vi "Setup Displacement.vi"(8 "error in (no error)":errorcluster, 10 "Model in":refnum<class "Model.lvclass">, 11 "Boot Loader in":refnum<class "Boot Loader.lvclass">) -> (0 "error out":errorcluster, 2 "Model out":refnum<class "Model.lvclass">, 3 "Boot Loader out":refnum<class "Boot Loader.lvclass">)   [LabVIEW 2016, in "Boot Loader.lvclass"]
uses:
  Boot Loader.lvclass
  Model/Model.lvclass
  Common_SerialProtocols/SerialProtocol/SerialReal/SerialReal.lvclass
  common_serialprotocols/Configuration/ProtocolParameters.ctl
  common_serialprotocols/Configuration/SerialMessageParameters.ctl
  Common_RT_DLRS1ADisplacementGauge/DLRS1ADisplacementGauge/DLRS1ADisplacementGauge.lvclass
  Model/Model.lvclass/Model.ctl
  Common_SerialProtocols/SerialProtocols.lvlib
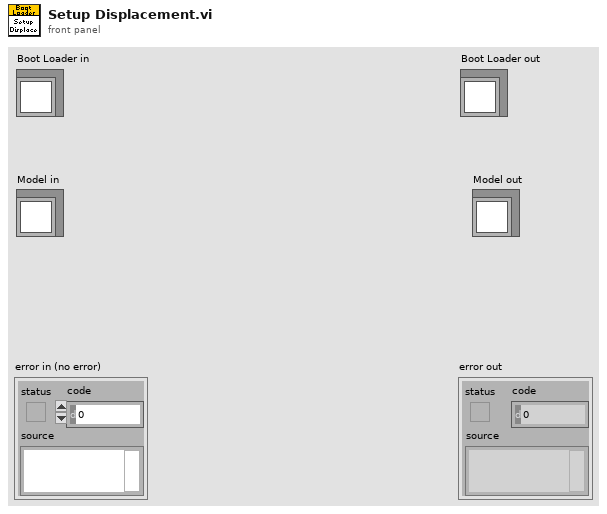
[diagram p1: front panel]
types:
  T1 = typedef "SerialProtocols.lvlib/SerialMessageParameters.ctl" = cluster{"Byte Count":u32, "Enable Termination Character":bool, "Termination Char":u8}
  T2 = typedef "SerialProtocols.lvlib/ProtocolParameters.ctl" = cluster{"VISA resource name":refnum<visa-resource-name>, "Baud Rate":u32, "Data Bits":u16, "Parity":enum16{"None", "Odd", "Even", "Mark", "Space"}, "Flow Control":u16, "Stop Bits":u16, "Timeout (ms)":u32}
  T3 = typedef "HPMT_Typedefs.lvlib/SerialSettings.ctl" = cluster{"Baud Rate":u32, "Data Bits":u16, "Parity":enum16{"None", "Odd", "Even", "Mark", "Space"}, "Flow Control":u16, "Stop Bits":u16, "Timeout (ms)":u32, "Byte Count":u32, "Enable Termination Character":bool, "Termination Char":u8}
  T4 = typedef "HPMT_Typedefs.lvlib/ConnectionSettings.ctl" = cluster{"ILC Port":refnum<visa-resource-name>, "Displacment Port\n":refnum<visa-resource-name>}
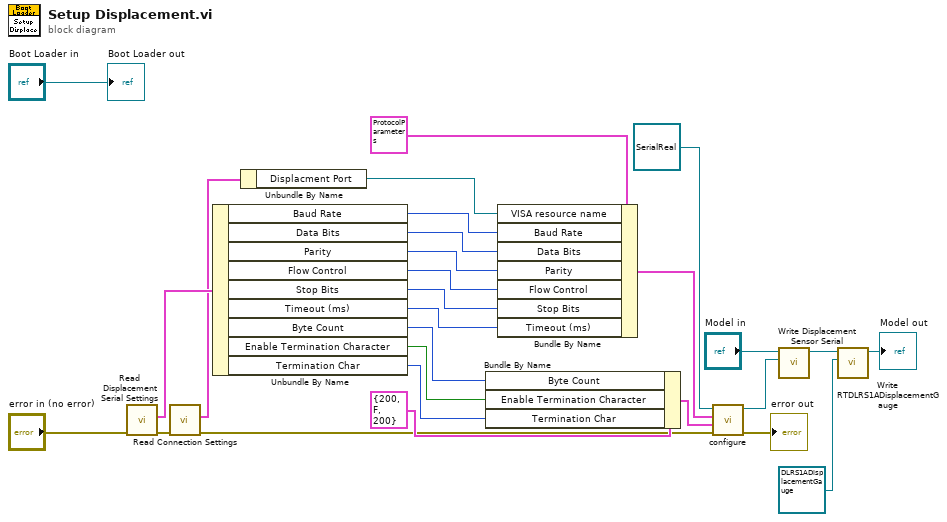
[diagram p0: block diagram]
diagram:
  n1 = call "Read Displacement Serial Settings.vi"("error in (no error)"="error in (no error)") -> ("error out"=w8:errorcluster, "Serial Settings"=w25:T3)  [unwired: 8 in, 1 out]
  n2 = call "Read Connection Settings.vi"("error in (no error)"=w8) -> ("error out"=w7:errorcluster, "Connection Settings"=w13:T4)  [unwired: 8 in, 1 out]
  n3 = Unbundle By Name(w25) -> ("Baud Rate"=w19:u32, "Data Bits"=w18:u16, "Parity"=w17:enum16{"None", "Odd", "Even", "Mark", "Space"}, "Flow Control"=w16:u16, "Stop Bits"=w15:u16, "Timeout (ms)"=w14:u32, "Byte Count"=w22:u32, "Enable Termination Character"=w21:bool, "Termination Char"=w20:u8)
  n4 = Unbundle By Name(w13) -> ("Displacment Port"=w12:refnum<visa-resource-name>)
  n5 = Bundle By Name(cluster=T1 {"Byte Count"=200, "Enable Termination Character"=FALSE, "Termination Char"=200} ("Serial Message Parameters"), "Byte Count"=w22, "Enable Termination Character"=w21, "Termination Char"=w20) -> (w10:T1)
  n6 = Bundle By Name(cluster=T2 {"VISA resource name"="", "Baud Rate"=9600, "Data Bits"=8, "Parity"=enum."None", "Flow Control"=0, "Stop Bits"=10, "Timeout (ms)"=10000} ("Protocol Parameters"), "VISA resource name"=w12, "Baud Rate"=w19, "Data Bits"=w18, "Parity"=w17, "Flow Control"=w16, "Stop Bits"=w15, "Timeout (ms)"=w14) -> (w11:T2)
  n7 = call-dynamic "configure.vi"("error in (no error)"=w7, "Serial Message Parameters"=w10, "Protocol Parameters"=w11, "SerialReal in"=refnum<class "SerialReal.lvclass"> refnum ("SerialProtocols.lvlib:SerialReal.lvclass")) -> ("error out"=→"error out":errorcluster, "SerialReal out"=w5:refnum<class "SerialReal.lvclass">)  [unwired: 6 in]
  n8 = call "Write Displacement Sensor Serial.vi"("SerialProtocols.lvlib:SerialReal.lvclass"=w5, "Model in"="Model in") -> ("Model out"=w4:refnum<class "Model.lvclass">)  [unwired: 9 in]
  n9 = call "Write RTDLRS1ADisplacementGauge.vi"("RTDLRS1ADisplacementGauge.lvlib:DLRS1ADisplacementGauge.lvclass"=refnum<class "DLRS1ADisplacementGauge.lvclass"> refnum, "Model in"=w4) -> ("Model out"=→"Model out":refnum<class "Model.lvclass">)  [unwired: 9 in]
  "Boot Loader out" <- "Boot Loader in"
